vi "ke2002_close.vi"(7 "thermo channel":T1={"type"=enum."COMET Tx5xx (ethernet)", "comment"="", "tag"="", "refresh"=5.0, "IP"="", "port"=502, "VISA"="", "last readout"=timestamp(0 s since 1904-01-01), "TCP ref"=refnum, "VISA sess"="", "idn"="", "press"=0.0, "RH"=0.0, "temp"=0.0, "pres cor"=[], "RH cor"=[], "temp cor"=[], "try left"=0, "failed"=FALSE, "RTD set"=[], "RTD inv"=[], "range"=0.0, "net mode"=enum."MODBUS", "try fail"=enum."Stop trying - return NaN", "timeout [s]"=0.0, "max retries"=0, "sim t [deg]"=0.0, "status"=0} {"status" items=["ok", "retry", "failed"]; "RTD inv" format="%.1f"; "RTD set" format="%.1f"; "temp cor" format="%.1f"; "RH cor" format="%.1f"; "pres cor" format="%.1f"; "refresh" min=0.1 max=1000.0 format="%.2f"}, 8 "error in":errorcluster, 11 "VISA in":refnum<visa-resource-name>) -> (0 "error out":errorcluster)   [LabVIEW 2020]
uses:
  thermo.ctl
  thermo_types.ctl
  Thermometer Fail Action.ctl
  <vilib>/Instr/_visa.llb/VISA GPIB Control REN Mode.ctl
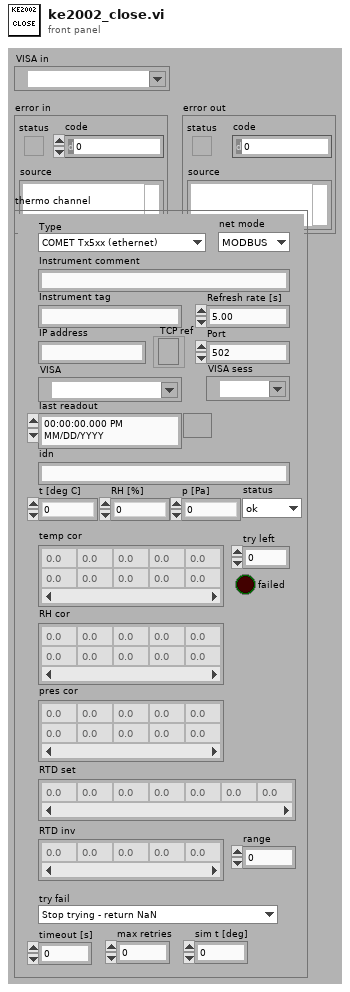
[diagram p1: front panel]
types:
  T1 = typedef "thermo.ctl" = cluster{"type":T2, "comment":string, "tag":string, "refresh":dbl, "IP":string, "port":u16, "VISA":refnum<visa-resource-name>, "last readout":timestamp, "TCP ref":refnum<k5>, "VISA sess":refnum<visa-resource-name>, "idn":string, "press":dbl, "RH":dbl, "temp":dbl, "pres cor":dbl[][], "RH cor":dbl[][], "temp cor":dbl[][], "try left":i32, "failed":bool, "RTD set":dbl[], "RTD inv":dbl[], "range":dbl, "net mode":enum16{"MODBUS", "HTTP"}, "try fail":T3, "timeout [s]":dbl, "max retries":i32, "sim t [deg]":dbl, "status":u16}
  T2 = typedef "thermo_types.ctl" = enum16{"Disabled", "Simulated", "COMET Tx5xx (ethernet)", "Keithley 2002 (GPIB) + RTD", "Agilent 344xx (GPIB) + RTD"}
  T3 = typedef "Thermometer Fail Action.ctl" = enum16{"Stop trying - keep last value", "Stop trying - return NaN", "Generate error - stop sweep"}
  T4 = typedef "VISA GPIB Control REN Mode.ctl" = u16
  T5 = cluster{"error":bool, "code":i32, "source":string}
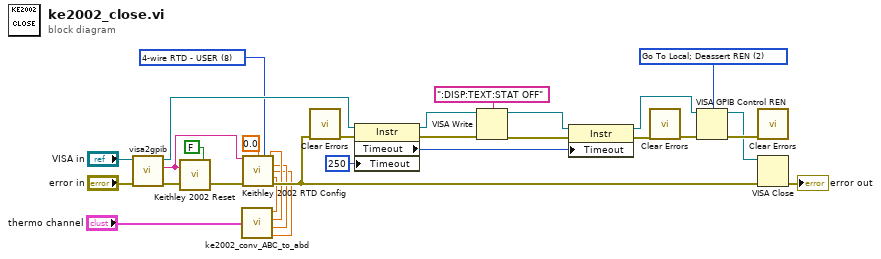
[diagram p0: block diagram]
diagram:
  w8 = u16 8 items=["2-wire RTD - PT385", "2-wire RTD - PT3916", "2-wire RTD - USER", "2-wire RTD - F100", "2-wire RTD - D100", "2-wire RTD - PT100", "4-wire RTD - PT385", "4-wire RTD - PT3916", "4-wire RTD - USER", "4-wire RTD - F100", "4-wire RTD - D100", "4-wire RTD - PT100"] ("transducer (2-W RTD-PT385:0)")
  w28 = T4 2 items=["Deassert REN", "Assert REN", "Go To Local; Deassert REN ", "Assert REN; Address Device", "Local Lockout (Addressed Devices)", "Local Lockout (This Device)", "Go To Local"] ("Mode")
  n1 = call "visa2gpib.vi"("error in"="error in", "VISA in"="VISA in") -> ("error out"=w24:errorcluster, "combined address"=w7:string, "VISA out"=w19:refnum<visa-resource-name>)  [unwired: 7 in]
  n2 = call "Keithley 2002 Reset.vi"("reset/preset"=FALSE, "error in"=w24, "GPIB address"=w7) -> ("error out"=w10:T5)
  n3 = call "ke2002_conv_ABC_to_abd.vi"("thermo"="thermo channel") -> ("R0"=w5:dbl, "alpha"=w4:dbl, "beta"=w3:dbl, "delta"=w2:dbl)
  n4 = call "Keithley 2002 RTD Config.vi"("GPIB address"=w7, "reference value (degs)"=0.0, "transducer (2-W RTD-PT385:0)"=w8, "alpha"=w4, "beta"=w3, "delta"=w2, "Rzero"=w5, "error in"=w10) -> ("error out"=w9:T5)  [unwired: 7 in]
  n5 = call <vilib>:"Clear Errors.vi"("error in (no error)"=w9) -> ("error out"=w20:errorcluster)  [unwired: 5 in, 1 out]
  n6 = property class="Instr"(reference=w19, error in=w20, "Timeout"=u32 250 ("timeout ms")) -> (reference out=w18:refnum<visa-resource-name>, error out=w17:errorcluster, "Timeout"=w13:u32)
  n7 = VISA Write(VISA resource name=w18, write buffer=":DISP:TEXT:STAT OFF", error in (no error)=w17) -> (VISA resource name out=w12:refnum<visa-resource-name>, error out=w15:errorcluster)  [unwired: 1 out]
  n8 = property class="Instr"(reference=w12, error in=w15, "Timeout"=w13) -> (reference out=w11:refnum<visa-resource-name>, error out=w14:errorcluster)
  n9 = call <vilib>:"Clear Errors.vi"("error in (no error)"=w14) -> ("error out"=w22:errorcluster)  [unwired: 5 in, 1 out]
  n10 = VISA GPIB Control REN(8:w22, 10:w28, 11:w11) -> (0:w30:errorcluster, 3:w29:refnum<visa-resource-name>)
  n11 = call <vilib>:"Clear Errors.vi"("error in (no error)"=w30) -> ()  [unwired: 5 in, 2 out]
  n12 = VISA Close(VISA resource name=w29, error in (no error)=w9) -> (error out=→"error out":errorcluster)
